vi "Client_NXT Copy.vi"   [LabVIEW 2011]
uses:
  <vilib>/NXT/Subs/MotorOutput.ctl
  <vilib>/NXT/Block Support/NXT_MessageMailbox.ctl
  <vilib>/NXT/Dual Mode Library/BT/BlueTooth_Read_num.vi
  <vilib>/NXT/Dual Mode Library/Display/drawNumber.vi
  <vilib>/NXT/Dual Mode Library/Motors/MotorOn.vi
  <vilib>/NXT/Dual Mode Library/BT/BlueTooth_Write_Float_toComputer.vi
panel:
  # "Deploy this code first.\n\nTarget to NXT."
types:
  T1 = typedef "MotorOutput.ctl" = u8
  T2 = typedef "NXT_MessageMailbox.ctl" = u8
  T3 = typedef "LVHSConnector.ctl" = cluster{"Hardware":string, "Flattened String":string}
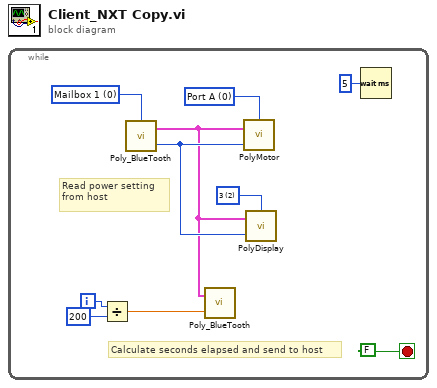
[diagram p0: block diagram]
diagram:
  n1 = while {
    i -> [w3]
    stop <- FALSE ("stop") stop-if-true
    w6 = i16 2 items=["1", "2", "3", "4", "5", "6", "7", "8"] ("Line")
    w9 = T1 0 items=["Port A"=0, "Port B"=1, "Port C"=2, "Ports A & B"=4, "Ports A & C"=5, "Ports B & C"=6, "All Ports"=3] ("Output Port (All Ports)")
    w10 = T2 0 items=["Mailbox 1", "Mailbox 2", "Mailbox 3", "Mailbox 4", "Mailbox 5", "Mailbox 6", "Mailbox 7", "Mailbox 8", "Mailbox 9", "Mailbox 10"] ("Mailbox")
    # "Read power setting from host"
    # "Calculate seconds elapsed and send to host"
    n2 = Divide(x=w3, y=200) -> (x/y=w1:dbl)
    n3 = call-poly <vilib>:"Poly_BlueTooth.vi"("Mailbox"=w10) -> ("Message"=w7:i32, "NXT"=w4:T3)  [unwired: 2 in]
    n4 = call-poly <vilib>:"Poly_BlueTooth.vi"("Message in"=w1, "NXT"=w4) -> ()  [unwired: 2 in, 1 out]
    n5 = call-poly <vilib>:"PolyMotor.vi"("Power (75)"=w7, "NXT"=w4, "Output Port (All Ports)"=w9) -> ()  [unwired: 1 in, 1 out]
    n6 = call-poly <vilib>:"PolyDisplay.vi"("number"=w7, "NXT"=w4, "Line"=w6) -> ()  [unwired: 1 in, 1 out]
    n7 = Wait (ms)(milliseconds to wait=u32 5) -> ()  [unwired: 1 out]
  }
